vi "Get Symbols.vi"(1 "Multichannel":T1 {"Filter"."IIR Filter Cluster"."Forward Coefficients" format="%.4f"; "Filter"."IIR Filter Cluster"."Reverse Coefficients" format="%.4f"}) -> (0 "Symbols":i32[](array[numeric]))   [LabVIEW 2020, in "Multichannel XCtl.xctl"]
uses:
  Multichannel XCtl.xctl
  Data.ctl
  Stimulus Channel XCtl/Stimulus Channel Data.ctl
  Waveform XCtl/Waveform Data.ctl
  Waveform XCtl/Waveform Enum.ctl
  Waveform VIs/Tone VIs/Tone Params.ctl
  Waveform VIs/Pulse Train VIs/Pulse Train Params.ctl
  Waveform VIs/Pulse Train VIs/Pulse Polarity.ctl
  Waveform VIs/Pulse Train VIs/PT-Continuous State.ctl
  Waveform VIs/Noise VIs/Noise Params.ctl
  Waveform VIs/File VIs/StimFile-Params.ctl
  Waveform VIs/FM Sweep VIs/FM Sweep Params.ctl
  Waveform VIs/Chirp Train VIs/Chirp Train.ctl
  Waveform VIs/Chirp Train VIs/Chirp Train Params.ctl
  Waveform VIs/Complex Tone VIs/CT-Params.ctl
  Waveform VIs/Complex Tone VIs/CT-Phase Enum.ctl
  Waveform VIs/Complex Tone VIs/CT-Runtime Data.ctl
  Waveform VIs/Moving Ripple VIs/Moving Ripple.ctl
  Waveform VIs/Moving Ripple VIs/Moving Ripple.Params.ctl
  Waveform VIs/Moving Ripple VIs/Moving Ripple.Data.ctl
  Filter XCtl/Filter Data.ctl
  Gate XCtl/Gate Data.ctl
  Level XCtl/Level Data.ctl
  Level XCtl/Level Units.ctl
  Filter XCtl/Filter XCtl.xctl
  Level XCtl/Level XCtl.xctl
  Gate XCtl/Gate Control.xctl
  Waveform XCtl/Waveform XCtl.xctl
  Stimulus Channel XCtl/Stimulus Channel.xctl
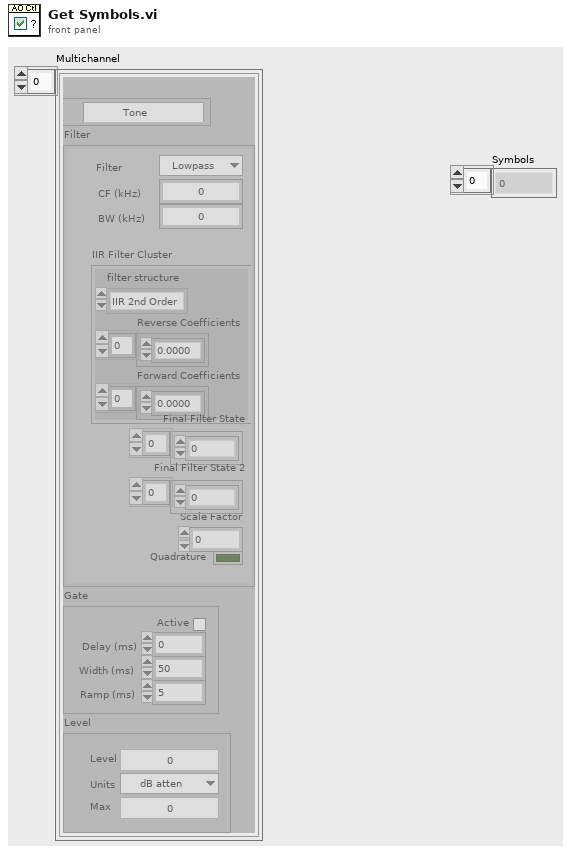
[diagram p1: front panel]
types:
  T1 = typedef "Multichannel XCtl.xctl/Data.ctl" = T2[]
  T2 = typedef "Stimulus Channel.xctl/Stimulus Channel Data.ctl" = cluster{"Waveform":T3, "Filter":T20, "Gate":T21, "Level":T22}
  T3 = typedef "Waveform XCtl.xctl/Waveform Data.ctl" = cluster{"Type":T4, "Tone":T5, "Pulse Train":T6, "Noise":T9, "File":T10, "FMSweep":T11, "Chirp Train":T12, "Complex Tone":cluster{"Params":T14, "Data":T16}, "Moving Ripple":T17}
  T4 = typedef "Waveform Enum.ctl" = enum16{"OFF", "Tone", "Noise", "Pulse Train", "File", "FM Sweep", "Chirp Train", "Complex Tone", "FM Tone", "Moving Ripple"}
  T5 = typedef "Tone Params.ctl" = cluster{"Frequency (kHz)":dbl, "Last Freq":dbl, "Last Phase":dbl}
  T6 = typedef "Pulse Train Params.ctl" = cluster{"Pulse width (us)":dbl, "Pulse rate (Hz)":dbl, "Gap (ms)":dbl, "Polarity":T7, "PT State":T8, "Asynch":bool}
  T7 = typedef "Pulse Polarity.ctl" = enum16{"POS", "NEG", "POS-NEG", "NEG-POS"}
  T8 = typedef "PT-Continuous State.ctl" = cluster{"Template":dbl[], "Nperiod":i32, "Index":i32, "Pulse Rate (Hz)":dbl, "Phase (cycles)":dbl, "Noff":i32}
  T9 = typedef "Noise Params.ctl" = cluster{"InvFilt":bool, "Noise":dbl[], "CurPt":i32, "Aweight":bool, "Seed":i32, "afile":path}
  T10 = typedef "StimFile-Params.ctl" = cluster{"Filename":path, "Signal":dbl[], "Channel":i32, "stream":bool, "offset":i32, "nreps":i32, "loops":i32, "Randomize":bool, "order":i32[], "Seed":i32, "Tokens":i32}
  T11 = typedef "FM Sweep Params.ctl" = cluster{"Rate (oct/s)":dbl, "Fmin (Hz)":dbl, "Fmax (Hz)":dbl, "Ramp (ms)":dbl, "Linear":bool}
  T12 = typedef "Chirp Train.ctl" = cluster{"Params":T13, "Data":cluster{"WF":dbl[]}}
  T13 = typedef "Chirp Train Params.ctl" = cluster{"Fmin (kHz)":dbl, "Fmax (kHz)":dbl, "Compensate":bool, "Duration (ms)":dbl}
  T14 = typedef "CT-Params.ctl" = cluster{"F0 (Hz)":dbl, "Band":cluster{"Flow (Hz)":dbl, "Fhigh (Hz)":dbl}, "Phase":T15, "Min F0 (Hz)":dbl, "Max F0 (Hz)":dbl, "ContinRandPhase":bool, "Max peak factor":dbl, "Max mod depth":dbl, "MinHarmNum":i32, "MaxHarmNum":i32, "Level Mode":enum16{"per component", "overall rms"}, "% jitter":dbl}
  T15 = typedef "CT-Phase Enum.ctl" = enum16{"Cosine", "Random", "Alternating"}
  T16 = typedef "CT-Runtime Data.ctl" = cluster{"Ncomp":i32, "MinHarm":i32, "Phase":dbl[], "Amplitude":dbl[], "Npts/frame":i32, "Last F0":dbl, "Fmin":dbl, "Fmax":dbl, "Lslope":dbl, "randphase":bool, "overall rms":bool, "fmult":dbl[], "jittered":bool}
  T17 = typedef "Moving Ripple.ctl" = cluster{"Params":T18, "Data":T19}
  T18 = typedef "Moving Ripple.Params.ctl" = cluster{"Fmin":dbl, "Fmax":dbl, "Density":dbl, "Velocity":dbl, "Depth":dbl, "Phase":dbl, "Comp/oct":i32}
  T19 = typedef "Moving Ripple.Data.ctl" = cluster{"Freq":dbl[], "A":dbl[], "phase":dbl[], "Phase":dbl}
  T20 = typedef "Filter XCtl.xctl/Filter Data.ctl" = cluster{"CF (kHz)":dbl, "BW (kHz)":dbl, "IIR Filter Cluster":cluster{"filter structure":enum32{"IIR 2nd Order", "IIR 4th Order"}, "Reverse Coefficients":dbl[], "Forward Coefficients":dbl[]}, "Final Filter State":dbl[], "Scale Factor":dbl, "Final Filter State 2":dbl[], "Quadrature":bool, "Type":enum16{"Lowpass", "Highpass", "Bandpass", "Bandstop", "OFF"}}
  T21 = typedef "Gate Control.xctl/Gate Data.ctl" = cluster{"Active":bool, "Delay (ms)":dbl, "Width (ms)":dbl, "Ramp (ms)":dbl}
  T22 = typedef "Level XCtl.xctl/Level Data.ctl" = cluster{"Level":dbl, "Units":T23, "Max":dbl, "Multiplier":dbl, "Cal File":path, "Cal":cluster{"Freq (Hz)":dbl[], "Mag (dB SPL)":dbl[], "Phase (deg)":dbl[]}}
  T23 = typedef "Level Units.ctl" = enum16{"dB atten", "dB SPL", "dB re 1 Vrms", "dB V/Hz½", "mW", "dB HL", "Volts", "dB mW"}
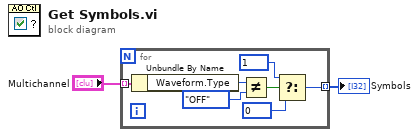
[diagram p0: block diagram]
diagram:
  n1 = for {
    tunnel: "Multichannel" -> [w9] mode=indexing
    tunnel: [w3] -> w1 mode=indexing
    n2 = Unbundle By Name(w9) -> ("Waveform.Type"=w8:T4)
    n3 = Not Equal?(x=w8, y=Waveform_Enum."OFF") -> (x != y?=w6:bool)
    n4 = Select(t=1, s=w6, f=0) -> (s? t:f=w3:i32)
  }
  "Symbols" <- w1
